vi "Test Base Clear Before Init Does Not Throw Error.vi"(8 "error in (no error)":errorcluster, 11 "Base Class Test In":refnum<class "Base Class Test.lvclass">) -> (0 "error out":errorcluster, 3 "Base Class Test Out":refnum<class "Base Class Test.lvclass">)   [LabVIEW 2020, in "Base Class Test.lvclass"]
uses:
  Base Class Test.lvclass
  C:/Program Files (x86)/National Instruments/LabVIEW 2020/vi.lib/Asteme/LUnit/Test Case.lvclass
  Base Class Test.lvclass/Base Class Test.ctl
  <vilib>/Asteme/LUnit/Test Case.lvclass/Test Case.ctl
  <vilib>/Asteme/LUnit/LUnit Assertion Result.lvclass/LUnit Assertion Result.ctl
  <vilib>/Asteme/LUnit/Palette/Pass.vi
  <vilib>/Asteme/LUnit/Palette/Fail.vi
  <vilib>/Asteme/LUnit/Set Assertion Type.vi
  <vilib>/Asteme/LUnit/Add test result.vi
  <vilib>/Asteme/LUnit/LUnit Write Passed.vi
  <vilib>/Asteme/LUnit/LUnit Get Test Case.vi
  <vilib>/Asteme/LUnit/LUnit Write Message.vi
  <vilib>/Asteme/LUnit/LUnit Write Description.vi
  <vilib>/Asteme/LUnit/LUnit Write Assertion Type.vi
  <vilib>/Asteme/LUnit/Read Test Case Name.vi
  <vilib>/Asteme/LUnit/Assertion Result/LUnit Get Test Name.vi
  Framework/Base/Base.lvclass
  <vilib>/Asteme/LUnit/LUnit Assertion Result.lvclass
  <vilib>/Asteme/LUnit/Test Case.lvclass
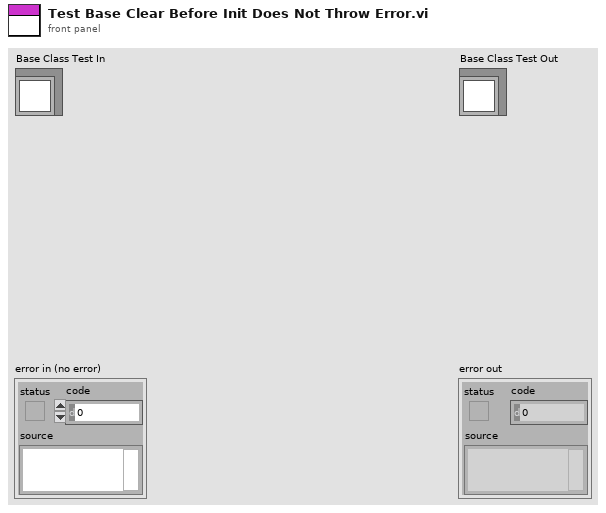
[diagram p1: front panel]
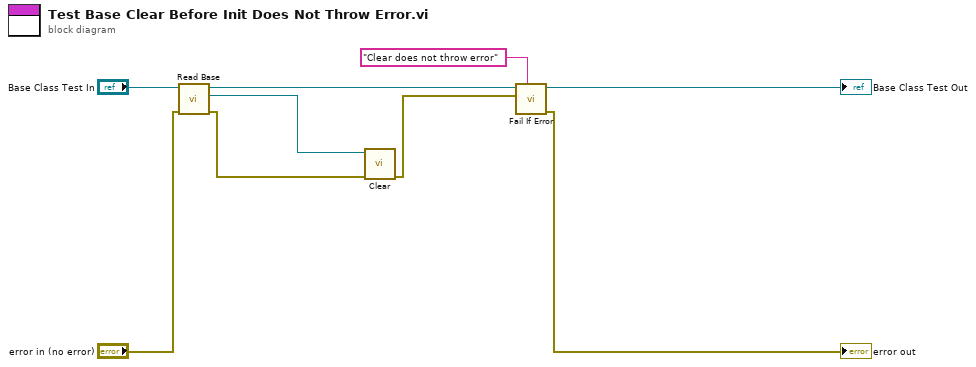
[diagram p0: block diagram]
diagram:
  n1 = call "Read Base.vi"("error in (no error)"="error in (no error)", "Base Class Test In"="Base Class Test In") -> ("error out"=w6:errorcluster, "Base.lvclass"=w7:refnum<class "Base.lvclass">, "Base Class Test Out"=w8:refnum<class "Base Class Test.lvclass">)  [unwired: 7 in]
  n2 = call-dynamic "Clear.vi"("error in (no error)"=w6, "Base In"=w7) -> ("error out"=w4:errorcluster)  [unwired: 8 in, 1 out]
  n3 = call <vilib>:"Fail If Error.vi"("Description"="Clear does not throw error", "Assert error"=w4, "Test Case In"=w8) -> ("error out"=→"error out":errorcluster, "Test Case Out"=→"Base Class Test Out":refnum<class "Base Class Test.lvclass">)  [unwired: 7 in]
